vi "Boost.vi"(11 "Flying Saucer in":refnum<class "Flying Saucer.lvclass">) -> (3 "Flying Saucer out":refnum<class "Flying Saucer.lvclass">)   [LabVIEW 2024, in "Flying Saucer.lvclass"]
doc: "MIT Licence\nCopyright (c) 2024 David Grollier"
uses:
  Flying Saucer.lvclass
  Type Def/Velocity.ctl
  Flying Saucer.lvclass/Flying Saucer.ctl
  Movable.lvclass
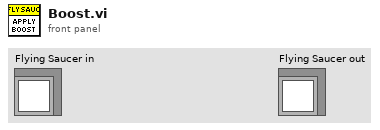
[diagram p1: front panel]
types:
  T1 = typedef "Velocity.ctl" = cluster{"Vx":dbl, "Vy":dbl}
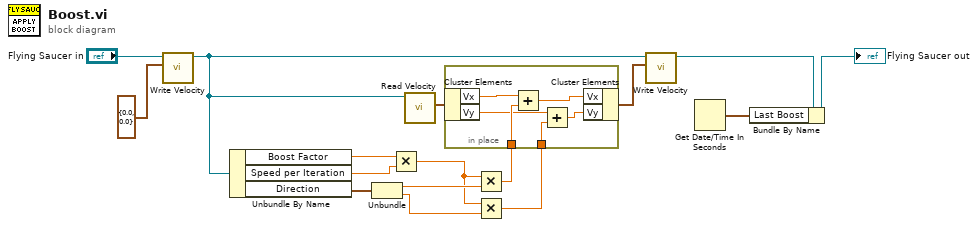
[diagram p0: block diagram]
diagram:
  n1 = call "Write Velocity.vi"("Velocity"=T1 {"Vx"=0.0, "Vy"=0.0}, "Movable in"="Flying Saucer in") -> ("Movable out"=w1:refnum<class "Flying Saucer.lvclass">)  [unwired: 9 in]
  n2 = Unbundle By Name(w1) -> ("Boost Factor"=w6:dbl, "Speed per Iteration"=w5:dbl, "Direction"=w9:T1)
  n3 = Unbundle(w9) -> ("Vx"=w15:dbl, "Vy"=w16:dbl)
  n4 = Multiply(x=w6, y=w5) -> (x*y=w4:dbl)
  n5 = call-dynamic "Read Velocity.vi"("Movable in"=w1) -> ("Velocity"=w12:T1)  [unwired: 10 in]
  n6 = Multiply(x=w4, y=w15) -> (x*y=w13:dbl)
  n7 = Multiply(x=w4, y=w16) -> (x*y=w14:dbl)
  n8 = in-place {
    in-place-border: w13 -> [w21]
    in-place-border: w14 -> [w18]
    n9 = in-place-cluster #1(w12) -> ("Vx"=w22:dbl, "Vy"=w19:dbl)
    n10 = Add(x=w22, y=w21) -> (x+y=w20:dbl)
    n11 = Add(x=w19, y=w18) -> (x+y=w17:dbl)
    n12 = in-place-cluster #1("Vx"=w20, "Vy"=w17) -> (w11:T1)
  }
  n13 = call "Write Velocity.vi"("Velocity"=w11, "Movable in"=w1) -> ("Movable out"=w10:refnum<class "Flying Saucer.lvclass">)  [unwired: 9 in]
  n14 = Get Date/Time In Seconds() -> (seconds since 1Jan1904=w7:timestamp)
  n15 = Bundle By Name(cluster=w10, "Last Boost"=w7) -> (→"Flying Saucer out":refnum<class "Flying Saucer.lvclass">)
